vi "RF_SetBitPath.vi"(7 "Path":path, 8 "error in (no error)":errorcluster) -> (0 "error out":errorcluster, 3 "return":i32)   [LabVIEW 2018]
uses:
  Common/Driver/rd.dll
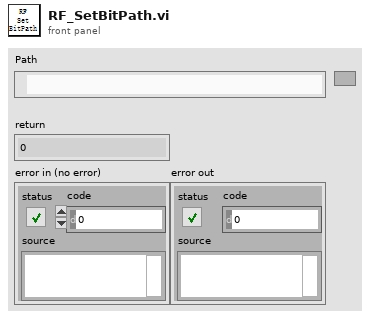
[diagram p1: front panel]
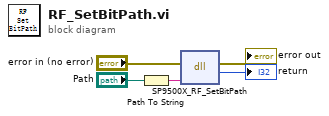
[diagram p0: block diagram]
diagram:
  n1 = Path To String(path="Path") -> (string=w1:string)
  n2 = dll-call lib="C:/rd/LabVIEW/Common/Driver/rd.dll" fn="SP9500X_RF_SetBitPath"(error in="error in (no error)", "Path"=w1) -> (error out=→"error out":errorcluster, "return"=→"return":i32)  [unwired: 3 in, 1 out]
